vi "labview_client2.vi"() -> ()   [LabVIEW 2019]
panel:
  out "Numeric":i32
  in  "stop":bool
  out "Python server reply (9 bytes) 3":string
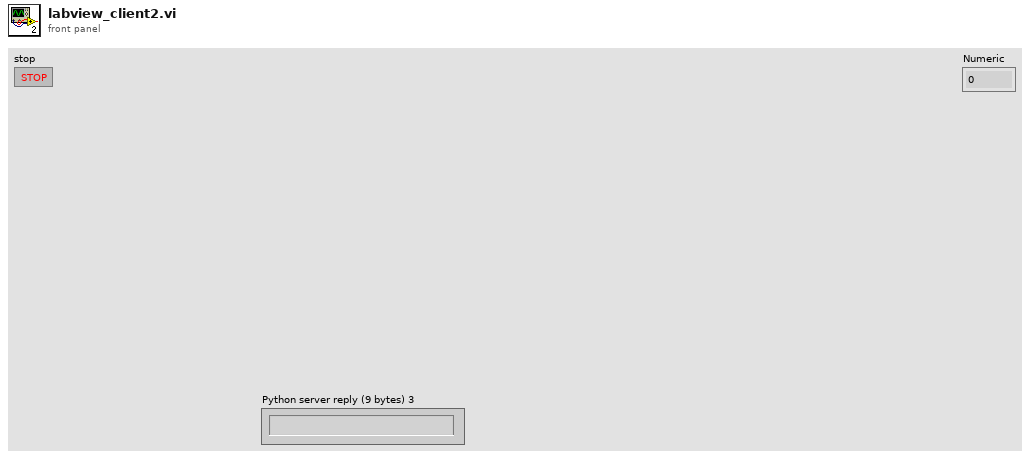
[diagram p1: front panel]
types:
  T1 = enum16{"Standard", "Buffered", "CRLF", "Immediate"}
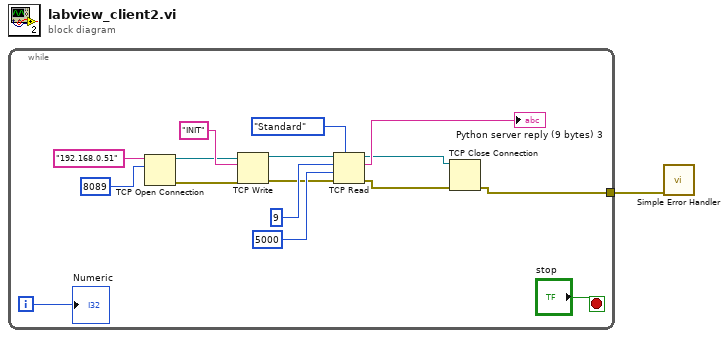
[diagram p0: block diagram]
diagram:
  n1 = while {
    tunnel: [w3] -> w1
    i -> [w2]
    stop <- "stop" stop-if-true
    n2 = TCP Open Connection(address="192.168.0.51", remote port or service name=u16 8089) -> (connection ID=w5:refnum<k5>, error out=w6:errorcluster)  [unwired: 3 in]
    n3 = TCP Write(connection ID=w5, data in="INIT", error in (no error)=w6) -> (connection ID out=w11:refnum<k5>, error out=w13:errorcluster)  [unwired: 1 in, 1 out]
    n4 = TCP Read(connection ID=w11, bytes to read=9, error in (no error)=w13, 7:T1."Standard" ("mode (standard)"), 9:5000 ("timeout ms (25000)")) -> (connection ID out=w9:refnum<k5>, data out=→"Python server reply (9 bytes) 3":string, error out=w10:errorcluster)
    n5 = TCP Close Connection(connection ID=w9, error in (no error)=w10) -> (error out=w3:errorcluster)  [unwired: 1 in, 1 out]
    "Numeric" <- w2
  }
  n6 = call <vilib>:"Simple Error Handler.vi"("error in (no error)"=w1) -> ()  [unwired: 4 in, 5 out]
